vi "LJcounter data file write.vi"(4 "Count":u32, 6 "Frequency":dbl format="%.2f", 8 "error in":errorcluster, 9 "seconds":ext format="%.3f", 10 "Write To File":bool, 11 "Data File":path=path "c:/temp/data.dat") -> (0 "error out":errorcluster)   [LabVIEW 2021]
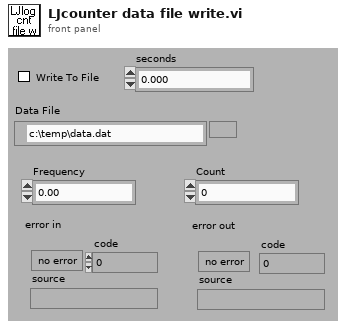
[diagram p1: front panel]
types:
  T1 = enum16{"open", "open or create", "create or replace", "create", "open (read only)"}
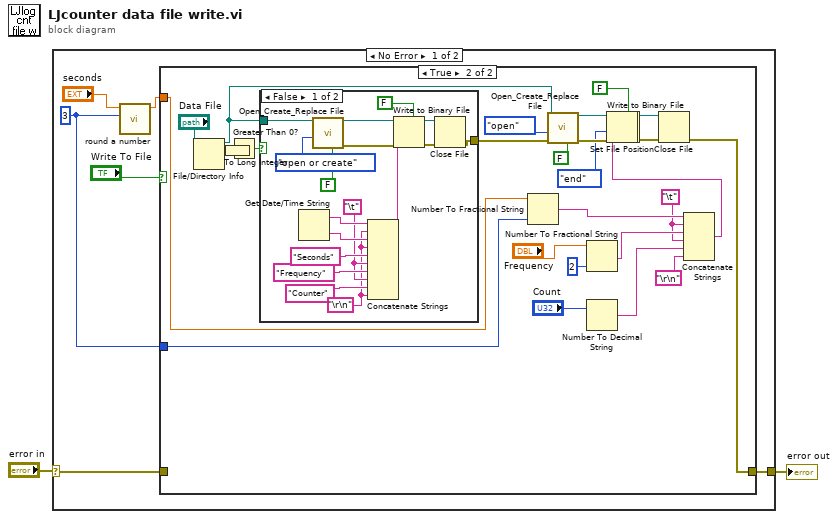
[diagram p0: block diagram]
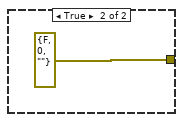
[diagram p3: hidden frame]
diagram:
  n1 = case shown="No Error" "error in" {
    selector: "error in" -> [w6 w56]
    tunnel: [w5 w56] -> w1
    frame No Error {
      w3 = 3 ("# decimal places to keep")
      n2 = call "round a number.vi"("# decimal places to keep"=w3, "Raw Value"="seconds") -> ("Rounded Value"=w7:dbl)  [unwired: 9 in]
      n3 = case shown="True" "Write To File" {
        tunnel: w7 -> [_ w27]
        tunnel: w6 -> [w9 _]
        tunnel: [w9 w22] -> w5
        tunnel: w3 -> [_ w14]
        frame False {
        }
        frame True {
          w17 = "\t"
          n4 = File/Directory Info(path="Data File") -> (path out=w29:path, size=w13:i64)  [unwired: 1 in, 5 out]
          n5 = To Long Integer(number=w13) -> (32bit integer=w37:i32)
          n6 = Greater Than 0?(x=w37) -> (x > 0?=w36:bool)
          n7 = case shown="False" w36 {
            tunnel: w29 -> [w54 _]
            tunnel: [w43 errorcluster {"status"=FALSE, "code"=0, "source"=""} ("error out")] -> w31
            frame False {
              w39 = "\r\n"
              w41 = "\t"
              n8 = Get Date/Time String() -> (date string=w50:string, time string=w49:string)  [unwired: 3 in]
              n9 = call <vilib>:"Open_Create_Replace File.vi"("advisory dialog? (display:T)"=FALSE, "function (open:0)"=T1."open or create", "file path"=w54) -> ("error out"=w47:errorcluster, "refnum"=w46:refnum<file>)  [unwired: 5 in, 2 out]
              n10 = Concatenate Strings(w50, w39, w49, w39, "Seconds" ("Substring"), w41, "Frequency" ("Substring"), w41, "Counter" ("Substring"), w39) -> (w48:string)
              n11 = Write to Binary File(file (use dialog)=w46, data=w48, error in=w47, 5:FALSE ("prepend array or string size? (T)")) -> (refnum out=w44:refnum<file>, error out=w45:errorcluster)  [unwired: 2 in, 1 out]
              n12 = Close File(refnum=w44, error in=w45) -> (error out=w43:errorcluster)  [unwired: 1 out]
            }
            frame True {
            }
          }
          n13 = Number To Fractional String(number=w27, precision (6)=w14) -> (F-format string=w25:string)  [unwired: 2 in]
          n14 = call <vilib>:"Open_Create_Replace File.vi"("advisory dialog? (display:T)"=FALSE, "error in (no error)"=w31, "function (open:0)"=T1."open", "file path"=w29) -> ("error out"=w32:errorcluster, "refnum"=w33:refnum<file>)  [unwired: 4 in, 2 out]
          n15 = Number To Fractional String(number="Frequency", precision (6)=i16 2) -> (F-format string=w18:string)  [unwired: 2 in]
          n16 = Number To Decimal String(number="Count") -> (decimal integer string=w16:string)  [unwired: 1 in]
          n17 = Set File Position(refnum=w33, from (0:start)=enum16{"start", "end", "current"}."end" ("pos mode (0:2)"), error in=w32) -> (refnum out=w12:refnum<file>, error out=w11:errorcluster)  [unwired: 1 in]
          n18 = Concatenate Strings(w25, w17, w18, w17, w16, "\r\n") -> (w24:string)
          n19 = Write to Binary File(file (use dialog)=w12, data=w24, error in=w11, 5:FALSE ("prepend array or string size? (T)")) -> (refnum out=w35:refnum<file>, error out=w34:errorcluster)  [unwired: 2 in, 1 out]
          n20 = Close File(refnum=w35, error in=w34) -> (error out=w22:errorcluster)  [unwired: 1 out]
        }
      }
    }
    frame Error {
    }
  }
  "error out" <- w1
